vi "Run_GCode.vi"(6 "Setup":T1, 8 "error in (no error)":errorcluster, 9 "Tool Refnum":refnum<vi>, 10 "VISA resource name in":refnum<visa-resource-name>, 11 "ListBox in":refnum<vi>) -> ()   [LabVIEW 2023]
uses:
  ShapekoGlobal.vi
panel:
  out "Timed out?":bool
  in  "Enable":bool
  out "Time elapsed":cluster{"second":i32, "minute":i32, "hour":i32}
  out "Done":i32(slide) scale=0.0..18795.0
  in  "Pause":bool
  out "Full Comm":string
  out "String in":string
  out "String out":string
  in  "Stop":bool
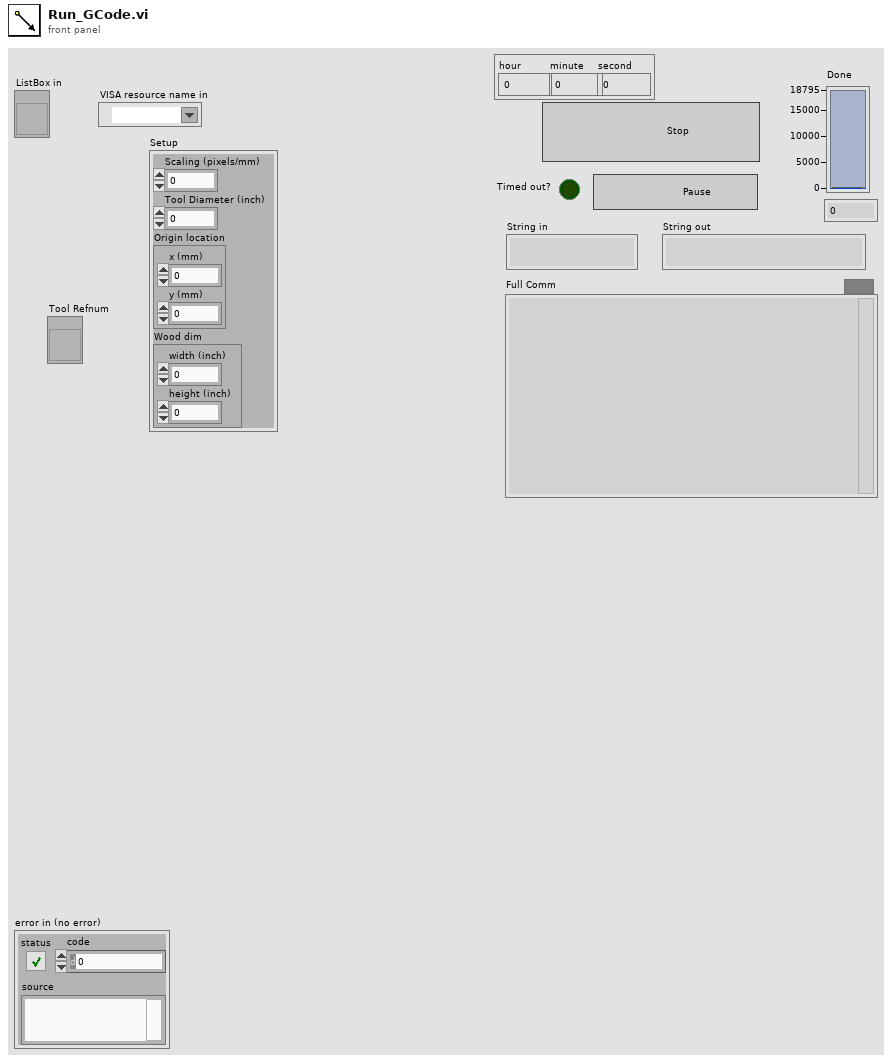
[diagram p1: front panel]
types:
  T1 = cluster{"Scaling (pixels/mm)":dbl, "Tool Diameter (inch)":dbl, "Origin location":cluster{"x (mm)":i16, "y (mm)":i16}, "Wood dim":cluster{"width (inch)":dbl, "height (inch)":dbl}}
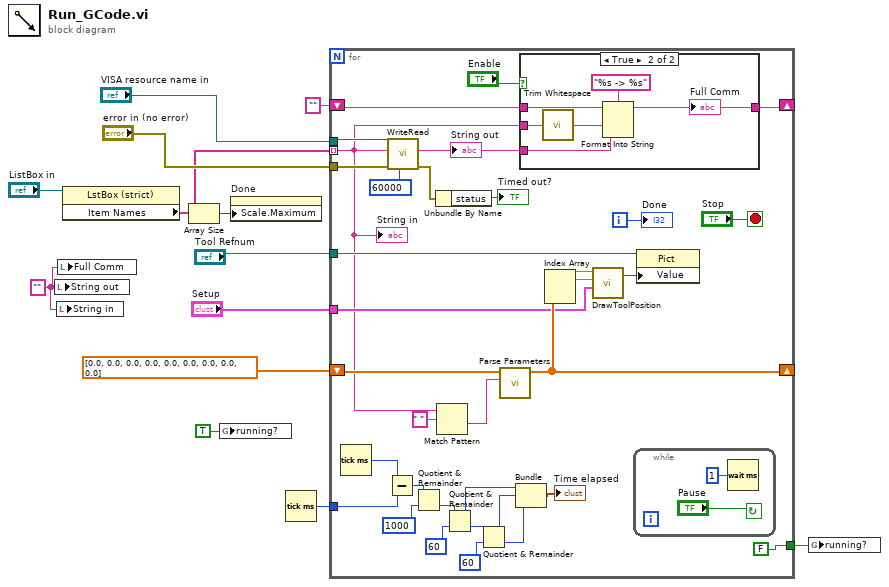
[diagram p0: block diagram]
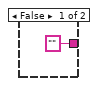
[diagram p2: hidden frame]
diagram:
  w4 = "" ("String out")
  n1 = local write "String out"(w4) -> ()
  n2 = local write "String in"(w4) -> ()
  n3 = local write "Full Comm"(w4) -> ()
  n4 = property on="Property Node" class="LstBox (strict)"(reference="ListBox in") -> ("Item Names"=w7:string[])  [unwired: 1 in, 2 out]
  n5 = Array Size(array=w7) -> (size(s)=w6:i32)
  n6 = global write "ShapekoGlobal.vi" "running?"(TRUE ("running?")) -> ()
  n7 = property on="Done" class="Slide (strict)"("Scale.Maximum"=w6) -> ()  [unwired: 2 in, 2 out]
  n8 = Tick Count (ms)() -> (millisecond timer value=w3:u32)
  n9 = for {
    tunnel: w7 -> [w34] mode=indexing
    tunnel: "VISA resource name in" -> [w47]
    tunnel: "error in (no error)" -> [w46]
    tunnel: "Tool Refnum" -> [w45]
    shift-right: [w40] -> _
    shift-left: dbl[] [0.0, 0.0, 0.0, 0.0, 0.0, 0.0, 0.0, 0.0, 0.0] -> [w41]
    tunnel: "Setup" -> [w37]
    shift-right: [w32] -> _
    shift-left: "" -> [w35]
    tunnel: w3 -> [w28]
    tunnel: [FALSE ("running?")] -> w1
    i -> [w31]
    stop <- "Stop" stop-if-true
    n10 = Tick Count (ms)() -> (millisecond timer value=w29:u32)
    n11 = Subtract(x=w29, y=w28) -> (x-y=w27:u32)
    n12 = call "WriteRead.vi"("Timeout (ms)"=60000, "error in (no error)"=w46, "String in"=w34, "VISA Refnum in"=w47) -> ("error out"=w19:errorcluster, "String out"=w33:string)  [unwired: 4 in, 2 out]
    "String out" <- w33
    n13 = Quotient & Remainder(x=w27, y=u32 1000) -> (floor(x/y)=w23:u32)  [unwired: 1 out]
    n14 = Unbundle By Name(w19) -> ("status"=→"Timed out?":bool)
    n15 = Match Pattern(string=w34, regular expression=" ") -> (after substring=w42:string)  [unwired: 1 in, 3 out]
    n16 = Quotient & Remainder(x=w23, y=u32 60) -> (x-y*floor(x/y)=w16:u32, floor(x/y)=w22:u32)
    n17 = Quotient & Remainder(x=w22, y=u32 60) -> (x-y*floor(x/y)=w15:u32, floor(x/y)=w14:u32)
    n18 = call "Parse Parameters.vi"("String"=w42, "Array in"=w41) -> ("Array out"=w40:dbl[])  [unwired: 9 in]
    n19 = Bundle(w16, w15, w14) -> (→"Time elapsed":cluster{u32, u32, u32})  [unwired: 1 in]
    n20 = case shown="True" "Enable" {
      tunnel: w35 -> [_ w53]
      tunnel: w34 -> [_ w52]
      tunnel: w33 -> [_ w50]
      tunnel: ["" w49] -> w32
      frame False {
      }
      frame True {
        n21 = call <vilib>:"Trim Whitespace.vi"("string"=w52) -> ("trimmed string"=w51:string)  [unwired: 1 in]
        n22 = Format Into String(format string="%s -> %s", initial string=w53, w51, w50) -> (resulting string=w49:string)  [unwired: 1 in, 1 out]
        "Full Comm" <- w49
      }
    }
    n23 = Index Array(array=w40) -> (element #1=w39:dbl, element #2=w38:dbl)  [unwired: 2 in]
    n24 = call "DrawToolPosition.vi"("Setup"=w37, "Y"=w38, "X"=w39) -> ("blob"=w44:picture)  [unwired: 8 in]
    n25 = while {
      stop <- "Pause" continue-if-true
      n26 = Wait (ms)(milliseconds to wait=u32 1) -> ()  [unwired: 1 out]
    }
    n27 = property on="Property Node" class="Pict"(reference=w45, "Value"=w44) -> ()  [unwired: 1 in, 2 out]
    "String in" <- w34
    "Done" <- w31
  }
  n28 = global write "ShapekoGlobal.vi" "running?"(w1) -> ()
